vi "ProcessH5Errors.vi"(4 "error in (no error)":errorcluster, 6 "Error code Offset":i32=8000, 7 "Error Stack in":T1[](array[typedef])) -> (0 "error out":errorcluster, 2 "Number of Errors":i32, 3 "Error Stack":T1[](array[typedef]))   [LabVIEW 2017]
uses:
  <vilib>/UPVI/lvhdf5/common.llb/HDF5 Error Cluster.ctl
panel:
  # "LVHDF5 Toolkit\nCopyright (c) 2005-2013 by Jason D. Sommerville\nCopyright (c) 2014 by UPVI, LLC.\n\nThis use and distribution of this file is governed by the terms found in \nLICENSE.txt distributed with this toolkit and installed at\n <user.lib>\\_lvhdf5\\LICENSE.txt"
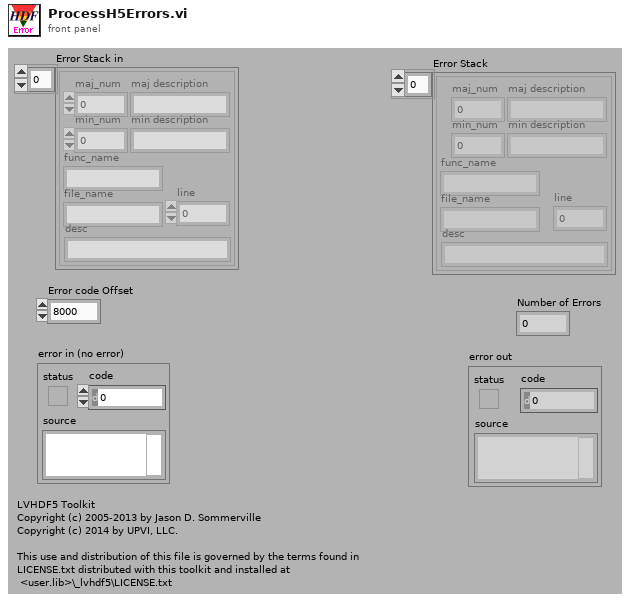
[diagram p1: front panel]
types:
  T1 = typedef "HDF5 Error Cluster.ctl" = cluster{"maj_num":i32, "min_num":i32, "func_name":string, "file_name":string, "line":u32, "desc":string, "maj description":string, "min description":string}
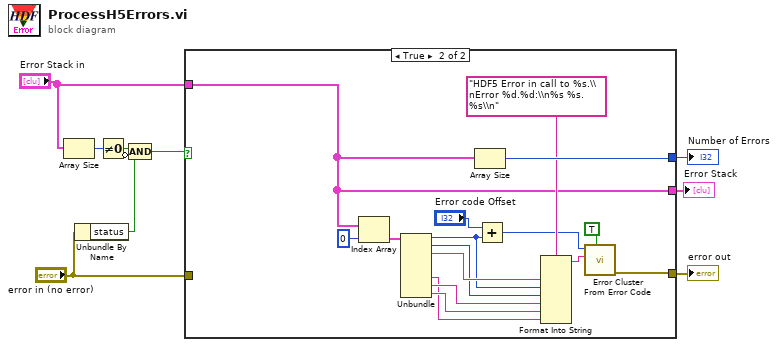
[diagram p0: block diagram]
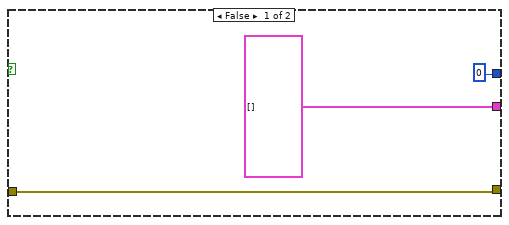
[diagram p2: hidden frame]
diagram:
  n1 = Array Size(array="Error Stack in") -> (size(s)=w3:i32)
  n2 = Unbundle By Name("error in (no error)") -> ("status"=w7:bool)
  n3 = Not Equal To 0?(x=w3) -> (x != 0?=w2:bool)
  n4 = Compound Arithmetic op=AND(w2, invert w7) -> (w6:bool)
  n5 = case shown="True" w6 {
    tunnel: [T1[] [] w13] -> w4
    tunnel: [w12 w26] -> w9
    tunnel: [0 ("num_errs") w28] -> w8
    tunnel: "error in (no error)" -> [w12 _]
    tunnel: "Error Stack in" -> [_ w13]
    frame False {
    }
    frame True {
      n6 = Index Array(array=w13, index=0) -> (element=w25:T1)
      n7 = Unbundle(w25) -> ("maj_num"=w21:i32, "min_num"=w18:i32, "func_name"=w22:string, "desc"=w15:string, "maj description"=w17:string, "min description"=w16:string)  [unwired: 2 out]
      n8 = Array Size(array=w13) -> (size(s)=w28:i32)
      n9 = Add(x="Error code Offset", y=w21) -> (x+y=w20:i32)
      n10 = Format Into String(format string="HDF5 Error in call to %s.\\nError %d.%d:\\n%s %s. %s\\n", w22, w21, w18, w17, w16, w15) -> (resulting string=w19:string)  [unwired: 2 in, 1 out]
      n11 = call <vilib>:"Error Cluster From Error Code.vi"("show call chain? (False)"=TRUE, "error message (\"\")"=w19, "error code (0)"=w20) -> ("error out"=w26:errorcluster)  [unwired: 6 in]
    }
  }
  "error out" <- w9
  "Number of Errors" <- w8
  "Error Stack" <- w4
